vi "Viavi - closeRefs.vi"(8 "error in (no error)":errorcluster {"code" format="Error %.0f"}, 11 "Viavi - strictRefs In":T1) -> (0 "error out":errorcluster {"code" format="Error %.0f"}, 3 "Viavi - strictRefs Out":T1)   [LabVIEW 2017]
uses:
  Controls/Viavi - objectRefs.ctl
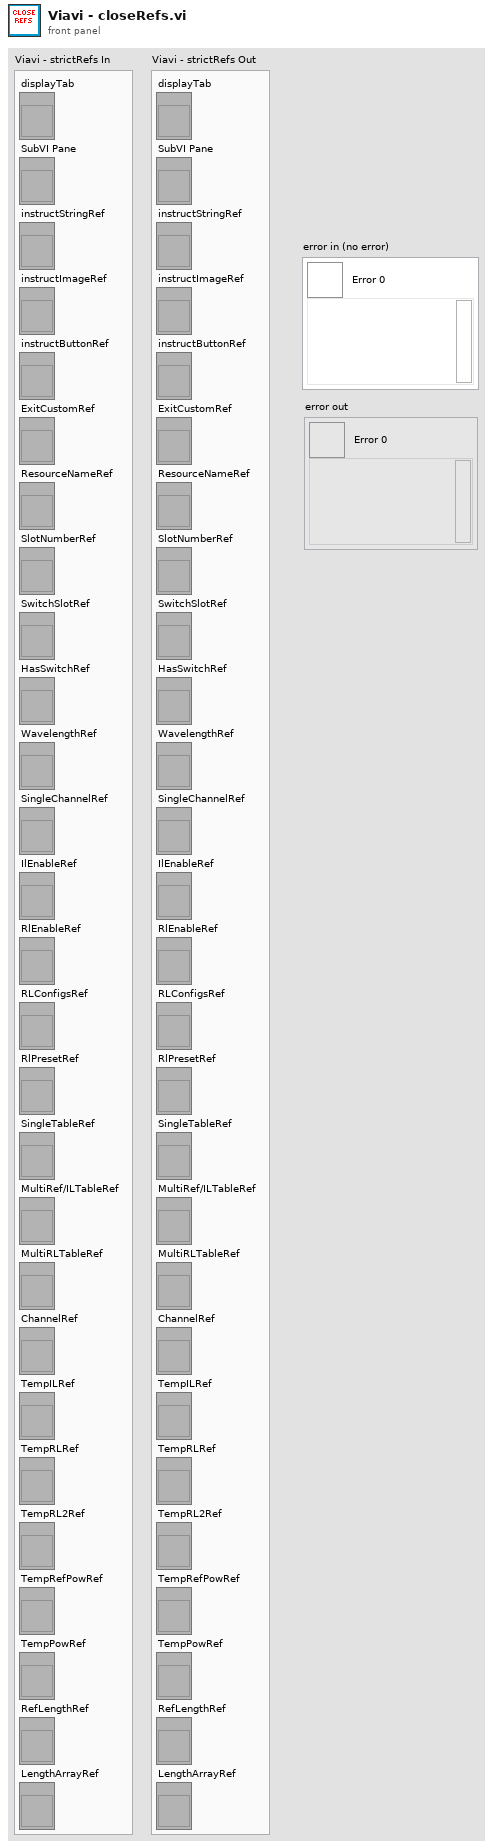
[diagram p1: front panel]
types:
  T1 = typedef "Viavi - objectRefs.ctl" = cluster{"displayTab":refnum<vi>, "SubVI Pane":refnum<vi>, "instructStringRef":refnum<vi>, "instructImageRef":refnum<vi>, "instructButtonRef":refnum<vi>, "ExitCustomRef":refnum<vi>, "ResourceNameRef":refnum<vi>, "SlotNumberRef":refnum<vi>, "SwitchSlotRef":refnum<vi>, "HasSwitchRef":refnum<vi>, "WavelengthRef":refnum<vi>, "SingleChannelRef":refnum<vi>, "IlEnableRef":refnum<vi>, "RlEnableRef":refnum<vi>, "RLConfigsRef":refnum<vi>, "RlPresetRef":refnum<vi>, "SingleTableRef":refnum<vi>, "MultiRef/ILTableRef":refnum<vi>, "MultiRLTableRef":refnum<vi>, "ChannelRef":refnum<vi>, "TempILRef":refnum<vi>, "TempRLRef":refnum<vi>, "TempRL2Ref":refnum<vi>, "TempRefPowRef":refnum<vi>, "TempPowRef":refnum<vi>, "RefLengthRef":refnum<vi>, "LengthArrayRef":refnum<vi>}
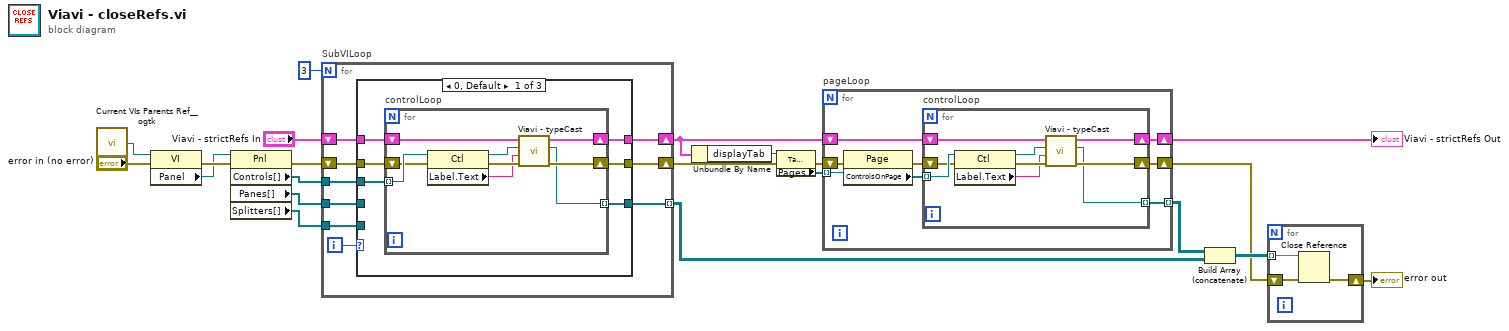
[diagram p0: block diagram]
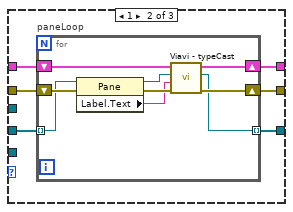
[diagram p2: hidden frame]
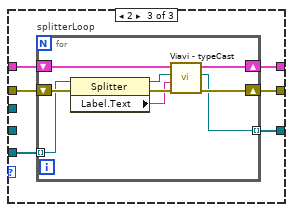
[diagram p3: hidden frame]
diagram:
  n1 = call <userlib>:"Current VIs Parents Ref__ogtk.vi"() -> ("Calling VI's Reference"=w13:refnum<vi>)  [unwired: 2 in]
  n2 = property class="VI"(reference=w13, error in="error in (no error)") -> (error out=w20:errorcluster, "Panel"=w18:refnum<vi>)  [unwired: 1 out]
  n3 = property class="Pnl"(reference=w18, error in=w20) -> (error out=w19:errorcluster, "Controls[]"=w14:refnum<vi>[], "Panes[]"=w16:refnum<vi>[], "Splitters[]"=w15:refnum<vi>[])  [unwired: 1 out]
  n4 = for "SubVILoop" {
    N: 3 -> [_]
    tunnel: w14 -> [w30]
    shift-right: [w28] -> w10
    shift-left: w19 -> [w29]
    shift-right: [w26] -> w7
    shift-left: "Viavi - strictRefs In" -> [w27]
    tunnel: w16 -> [w24]
    tunnel: w15 -> [w23]
    tunnel: [w22] -> w5 mode=indexing
    i -> [w25]
    n5 = case shown="0, Default" w25 {
      tunnel: w30 -> [w36 _ _]
      tunnel: w29 -> [w35 w51 w66]
      tunnel: [w34 w50 w65] -> w28
      tunnel: w27 -> [w33 w49 w64]
      tunnel: [w32 w48 w63] -> w26
      tunnel: w24 -> [_ w47 _]
      tunnel: w23 -> [_ _ w62]
      tunnel: [w31 w46 w61] -> w22
      frame 0, Default {
        n6 = for "controlLoop" {
          tunnel: w36 -> [w45] mode=indexing
          shift-right: [w39] -> w34
          shift-left: w35 -> [w44]
          shift-right: [w40] -> w32
          shift-left: w33 -> [w43]
          tunnel: [w37] -> w31 mode=indexing
          n7 = property class="Ctl"(reference=w45, error in=w44) -> (reference out=w42:refnum<vi>, error out=w41:errorcluster, "Label.Text"=w38:string)
          n8 = call "Viavi - typeCast.vi"("error in"=w41, "Label Name"=w38, "Input Refnum"=w42, "Viavi - strictRefs In"=w43) -> ("error out"=w39:errorcluster, "Cast Refnum"=w37:refnum<vi>, "Viavi - strictRefs Out"=w40:T1)  [unwired: 4 in, 1 out]
        }
      }
      frame 1 {
        n9 = for "paneLoop" {
          shift-right: [w55] -> w50
          shift-left: w51 -> [w60]
          shift-right: [w56] -> w48
          shift-left: w49 -> [w59]
          tunnel: w47 -> [w53] mode=indexing
          tunnel: [w52] -> w46 mode=indexing
          n10 = property class="Pane"(reference=w53, error in=w60) -> (reference out=w58:refnum<vi>, error out=w57:errorcluster, "Label.Text"=w54:string)
          n11 = call "Viavi - typeCast.vi"("error in"=w57, "Label Name"=w54, "Input Refnum"=w58, "Viavi - strictRefs In"=w59) -> ("error out"=w55:errorcluster, "Cast Refnum"=w52:refnum<vi>, "Viavi - strictRefs Out"=w56:T1)  [unwired: 4 in, 1 out]
        }
      }
      frame 2 {
        n12 = for "splitterLoop" {
          shift-right: [w70] -> w65
          shift-left: w66 -> [w75]
          shift-right: [w71] -> w63
          shift-left: w64 -> [w74]
          tunnel: w62 -> [w68] mode=indexing
          tunnel: [w67] -> w61 mode=indexing
          n13 = property class="Splitter"(reference=w68, error in=w75) -> (reference out=w73:refnum<vi>, error out=w72:errorcluster, "Label.Text"=w69:string)
          n14 = call "Viavi - typeCast.vi"("error in"=w72, "Label Name"=w69, "Input Refnum"=w73, "Viavi - strictRefs In"=w74) -> ("error out"=w70:errorcluster, "Cast Refnum"=w67:refnum<vi>, "Viavi - strictRefs Out"=w71:T1)  [unwired: 4 in, 1 out]
        }
      }
    }
  }
  n15 = Unbundle By Name(w7) -> ("displayTab"=w11:refnum<vi>)
  n16 = property class="TabCtl (strict)"(reference=w11, error in=w10) -> (error out=w8:errorcluster, "Pages"=w9:refnum<vi>[])  [unwired: 1 out]
  n17 = for "pageLoop" {
    tunnel: w9 -> [w82] mode=indexing
    shift-right: [w78] -> w2
    shift-left: w8 -> [w83]
    shift-right: [w77] -> w6
    shift-left: w7 -> [w79]
    tunnel: [w76] -> w4 mode=indexing
    n18 = property class="Page"(reference=w82, error in=w83) -> (error out=w81:errorcluster, "ControlsOnPage"=w80:refnum<vi>[])  [unwired: 1 out]
    n19 = for "controlLoop" {
      tunnel: w80 -> [w92] mode=indexing
      shift-right: [w86] -> w78
      shift-left: w81 -> [w91]
      shift-right: [w87] -> w77
      shift-left: w79 -> [w90]
      tunnel: [w84] -> w76 mode=indexing
      n20 = property class="Ctl"(reference=w92, error in=w91) -> (reference out=w89:refnum<vi>, error out=w88:errorcluster, "Label.Text"=w85:string)
      n21 = call "Viavi - typeCast.vi"("error in"=w88, "Label Name"=w85, "Input Refnum"=w89, "Viavi - strictRefs In"=w90) -> ("error out"=w86:errorcluster, "Cast Refnum"=w84:refnum<vi>, "Viavi - strictRefs Out"=w87:T1)  [unwired: 4 in, 1 out]
    }
  }
  "Viavi - strictRefs Out" <- w6
  n22 = Build Array (concatenate)(w4, w5) -> (w3:refnum<vi>[][])
  n23 = for {
    tunnel: w3 -> [w95] mode=indexing
    shift-right: [w93] -> w1
    shift-left: w2 -> [w94]
    n24 = Close Reference(reference=w95, error in (no error)=w94) -> (error out=w93:errorcluster)
  }
  "error out" <- w1
